vi "CRYAPI WSYSTEM MAIN.vi"(8 "sData":string, 9 "pVIF":refnum<vi>, 10 "sOption":string, 11 "sAction":string) -> (0 "bResult":bool=TRUE, 1 "pVIF_Out":refnum<vi>, 2 "sData_Out":string, 3 "tFrame_Out":T2)   [LabVIEW 2013]
uses:
  <vilib>/Utility/miscctls.llb/LVRectTypeDef.ctl
  CRYMain Sub Window Global.vi
  DataView/VIEW/CRYView Global.vi
  CRYProject/CRYProject Editor Global.vi
  DataView/VIEW/CRYNew View Global.vi
  CRYCurveLibrary/Global/CRYCurve Library Global.vi
  CRYStepSetup/CRYStepSetup Global.vi
  user32.dll
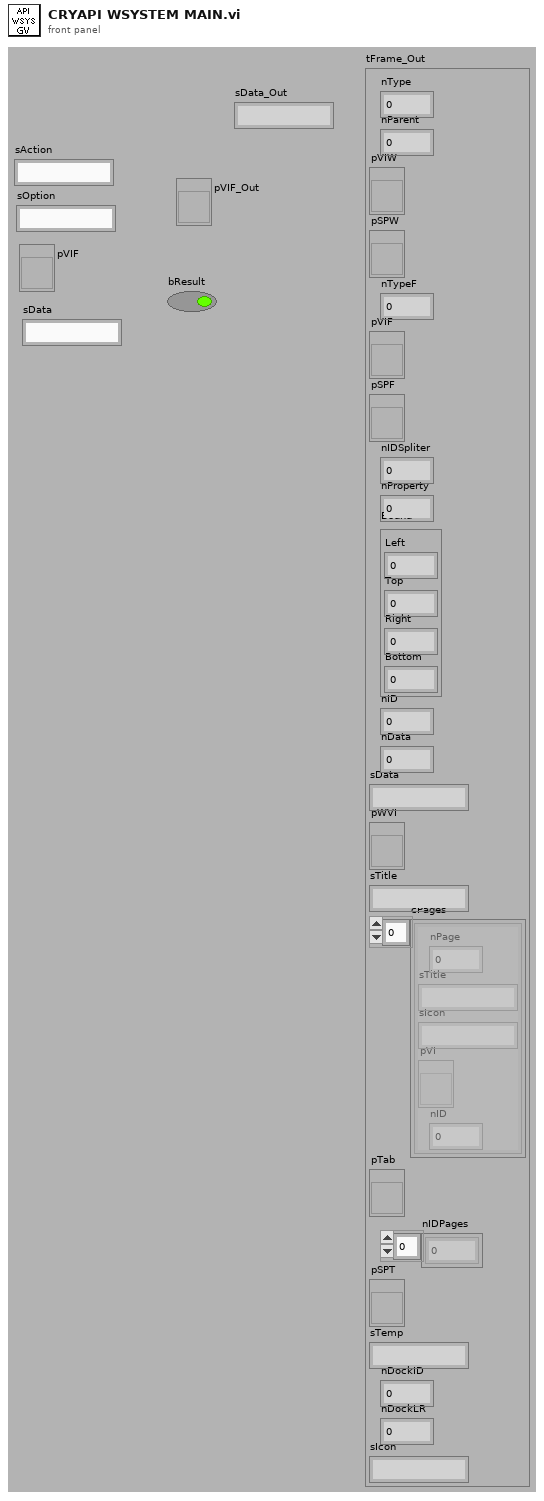
[diagram p1: front panel]
types:
  T1 = typedef "LVRectTypeDef.ctl" = cluster{"Left":i16, "Top":i16, "Right":i16, "Bottom":i16}
  T2 = cluster{"nType":i32, "nParent":i32, "pVIW":refnum<vi>, "pSPW":refnum<vi>, "nTypeF":i32, "pVIF":refnum<vi>, "pSPF":refnum<vi>, "nIDSpliter":i32, "nProperty":i32, "Bound":T1, "nID":i32, "nData":i32, "sData":string, "pWVI":refnum<vi>, "sTitle":string, "cPages":cluster{"nPage":i32, "sTitle":string, "sIcon":string, "pVI":refnum<vi>, "nID":i32}[], "pTab":refnum<vi>, "nIDPages":i32[], "pSPT":refnum<vi>, "sTemp":string, "nDockID":i32, "nDockLR":i32, "sIcon":string}
  T3 = enum32{"Invalid", "Standard", "Closed", "Hidden", "Minimized", "Maximized"}
  T4 = cluster{"nID":i32[], "Frame":cluster{"nType":i32, "nParent":i32, "pVIW":refnum<vi>, "pSPW":refnum<vi>, "nTypeF":i32, "pVIF":refnum<vi>, "pSPF":refnum<vi>, "nIDSpliter":i32, "nProperty":i32, "Bound":T1, "nID":i32, "nData":i32, "sData":string, "pWVI":refnum<vi>, "sTitle":string, "cPages":cluster{"nPage":i32, "sTitle":string, "sIcon":string, "pVI":refnum<vi>, "nID":i32}[], "pTab":refnum<vi>, "nIDPages":i32[], "pSPT":refnum<vi>, "sTemp":string, "nDockID":i32, "nDockLR":i32, "sIcon":string}[]}
  T5 = cluster{"nType":i32, "nParent":i32, "pVIW":refnum<vi>, "pSPW":refnum<vi>, "nTypeF":i32, "pVIF":refnum<vi>, "pSPF":refnum<vi>, "nIDSpliter":i32, "nProperty":i32, "Bound":T1, "nID":i32, "nData":i32, "sData":string, "pWVI":refnum<vi>, "sTitle":string, "cPages":cluster{"nPage":i32, "sTitle":string, "sIcon":string, "pVI":refnum<vi>, "nID":i32}[], "pTab":refnum<vi>, "nIDPages":i32[], "pSPT":refnum<vi>, "sTemp":string, "nDockID":i32, "nDockLR":i32, "sIcon":string}[]
  T6 = cluster{"Type Name":string, "Data Name":string, "Probe VIRef Number":i32, "Probe VIRef":refnum<vi>}[]
  T7 = cluster{"CLOSE_HIDE":i32, "CLOSE_CLOSE":i32, "DOCK_ENABLE":i32, "DOCK_DISABLE":i32, "FOCUS_SHOW":i32, "FOCUS_HIDE":i32}
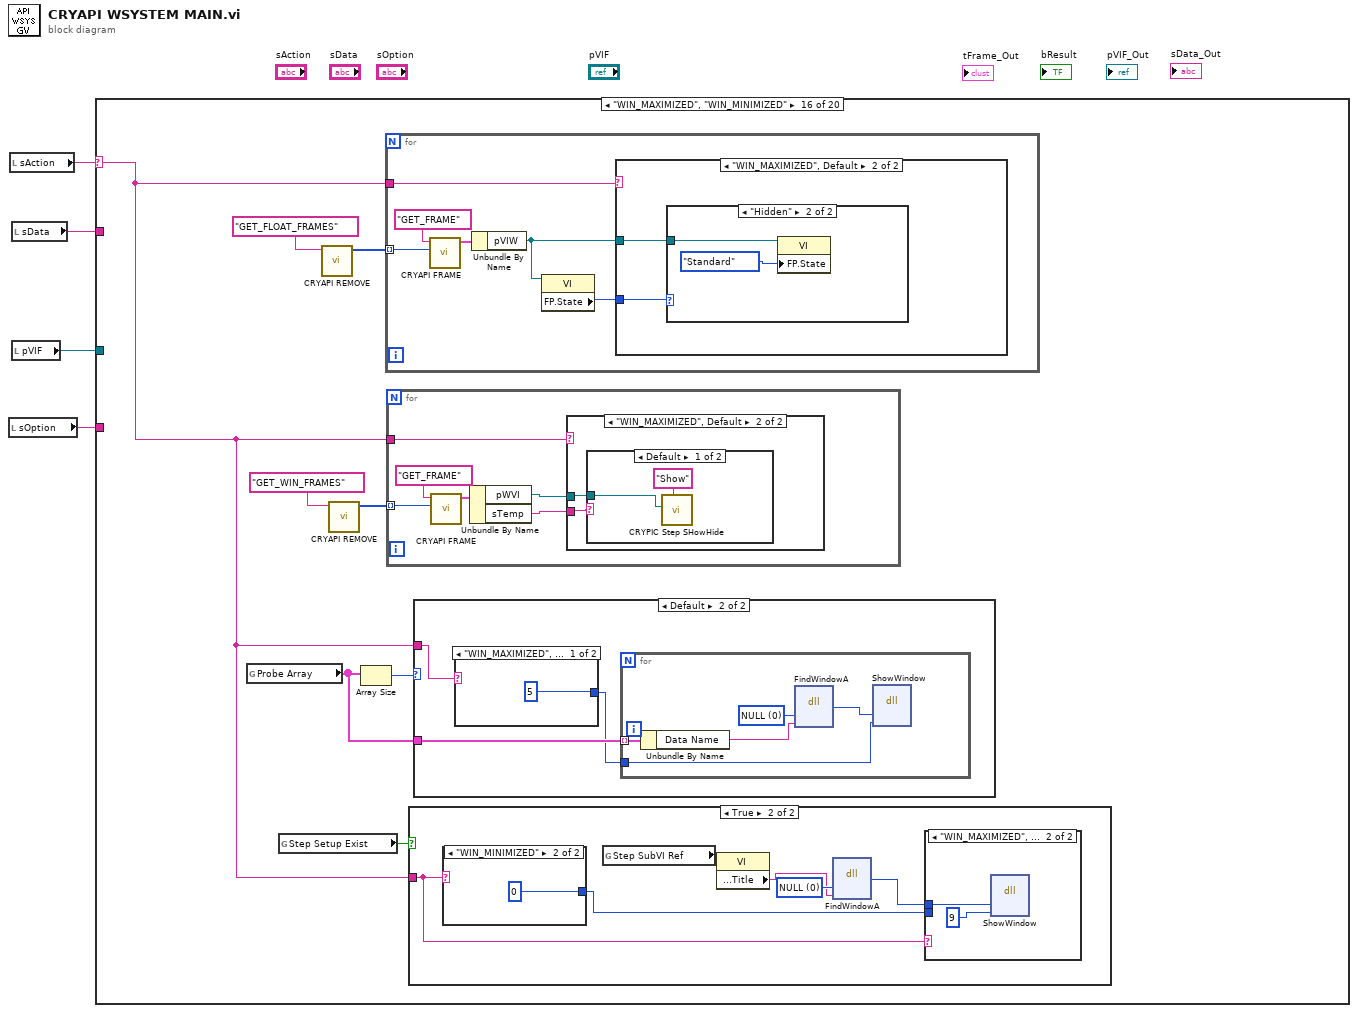
[diagram p0: block diagram]
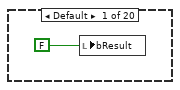
[diagram p2: hidden frame]
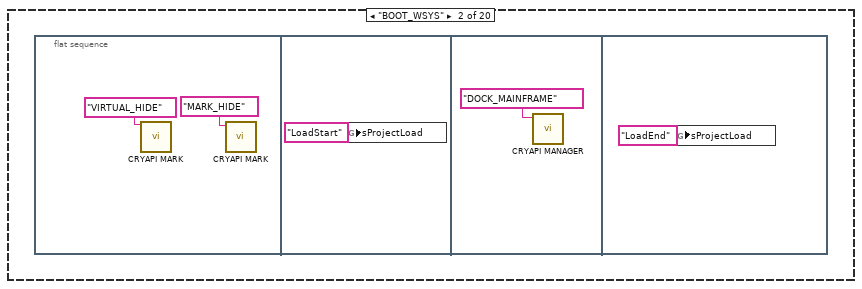
[diagram p3: hidden frame]
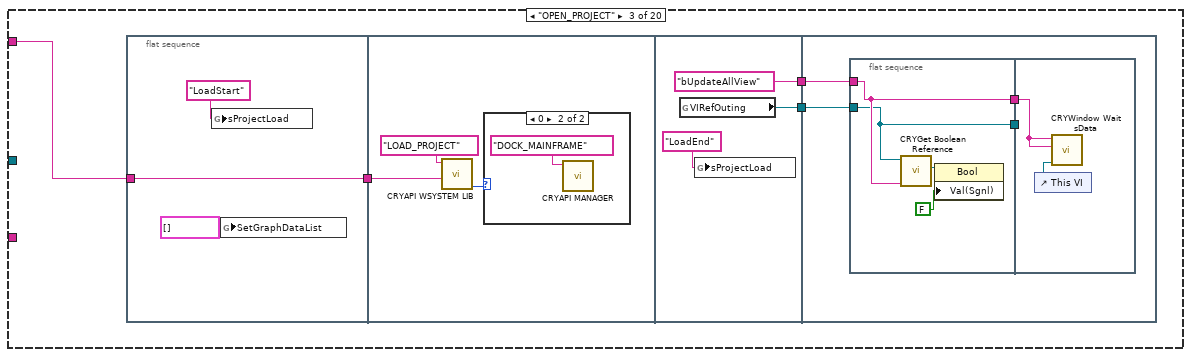
[diagram p4: hidden frame]
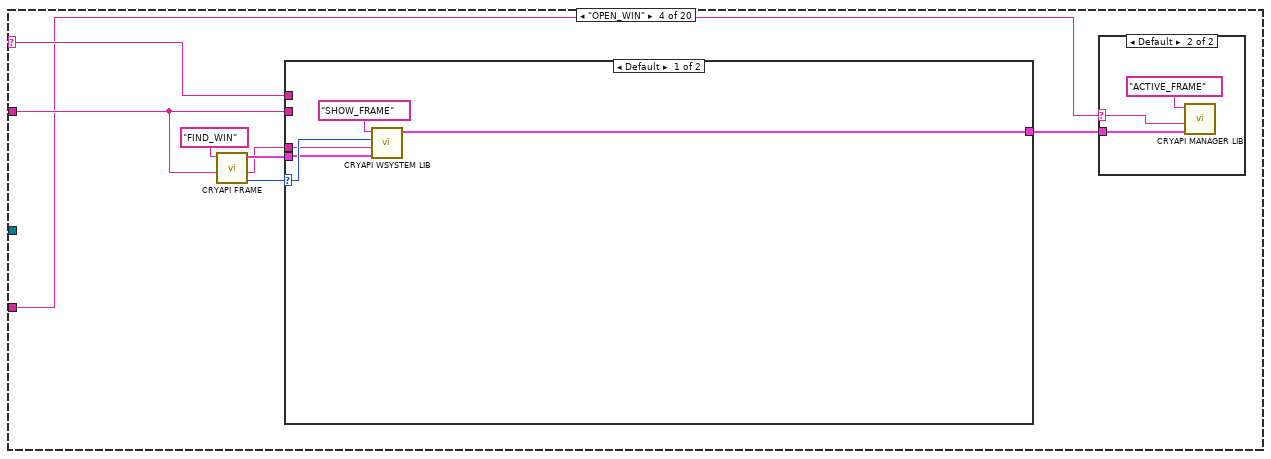
[diagram p6: hidden frame]
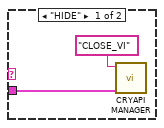
[diagram p7: hidden frame]
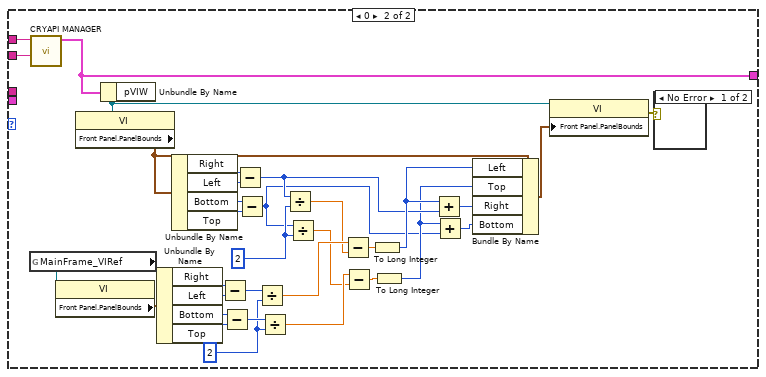
[diagram p8: hidden frame]
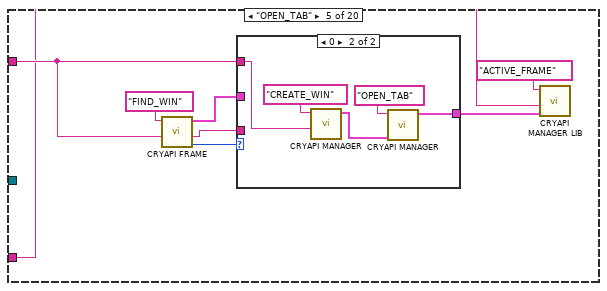
[diagram p10: hidden frame]
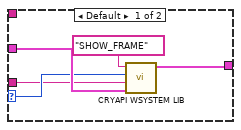
[diagram p11: hidden frame]
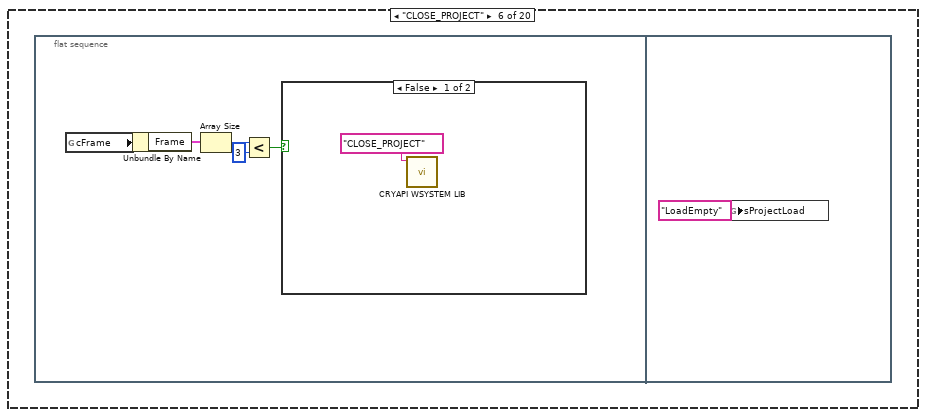
[diagram p12: hidden frame]
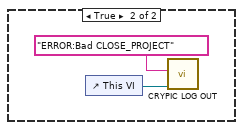
[diagram p13: hidden frame]
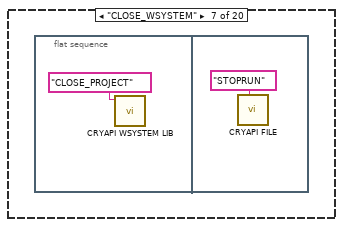
[diagram p14: hidden frame]
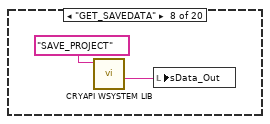
[diagram p15: hidden frame]
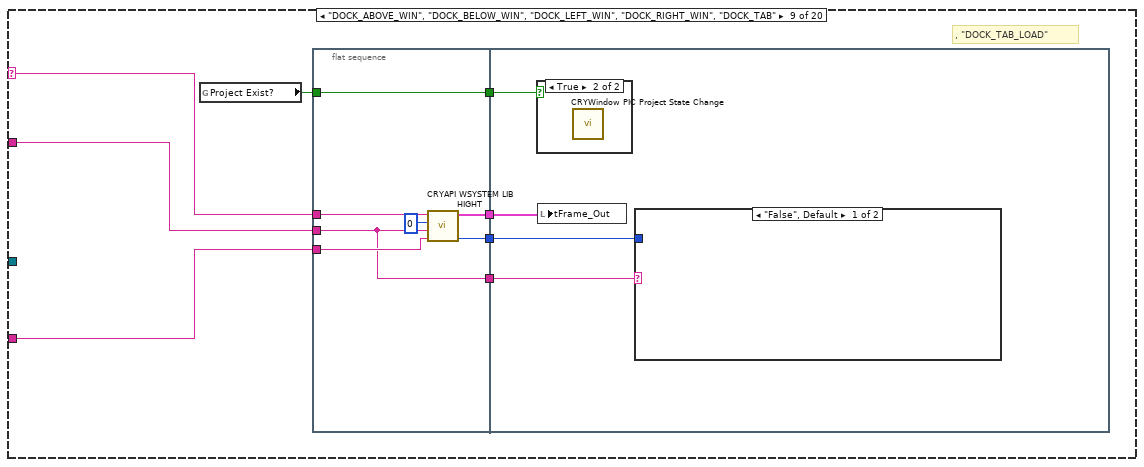
[diagram p16: hidden frame]
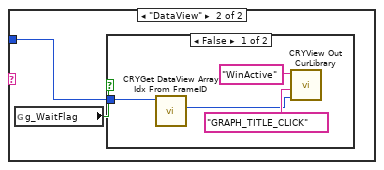
[diagram p17: hidden frame]
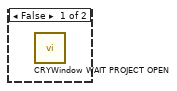
[diagram p19: hidden frame]
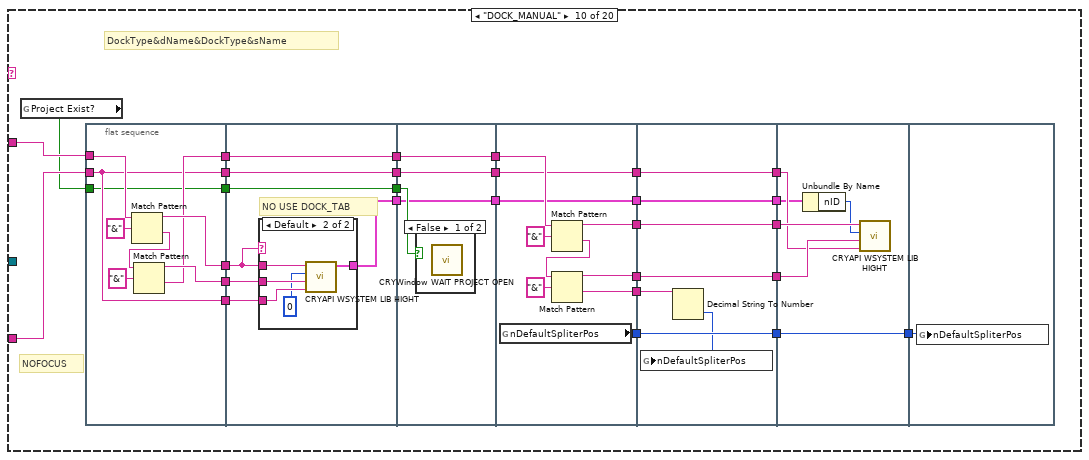
[diagram p20: hidden frame]
diagram:
  n1 = local read "sOption"() -> (w1:string)
  n2 = local read "sAction"() -> (w4:string)
  n3 = local read "sData"() -> (w3:string)
  n4 = local read "pVIF"() -> (w2:refnum<vi>)
  n5 = case shown="\"WIN_MAXIMIZED\", \"WIN_MINIMIZED\"" w4 {
    selector: w4 -> [_ _ _ w42 _ _ _ _ w122 _ _ w234 _ _ w292 w310 _ _ _ w422]
    tunnel: w3 -> [_ _ w14 w40 w90 _ _ _ w124 w165 _ w232 w275 w286 _ _ w375 w401 w420 _]
    tunnel: w2 -> [_ _ _ _ _ _ _ _ _ _ _ w241 _ _ _ _ _ _ _ _]
    tunnel: w1 -> [_ _ _ w35 w86 _ _ _ w123 w164 _ w230 w274 _ _ _ _ _ _ _]
    frame Default {
      n6 = local write "bResult"(FALSE) -> ()
    }
    frame "BOOT_WSYS" {
      n7 = flat-sequence {
        frame #0 {
          n8 = call "CRYAPI MARK.vi"("sAction"="VIRTUAL_HIDE") -> ()  [unwired: 3 in, 7 out]
          n9 = call "CRYAPI MARK.vi"("sAction"="MARK_HIDE") -> ()  [unwired: 3 in, 7 out]
        }
        frame #1 {
          n10 = global write "CRYMain Sub Window Global.vi" "sProjectLoad"("LoadStart" ("sProjectLoad")) -> ()
        }
        frame #2 {
          n11 = call "CRYAPI MANAGER.vi"("sAction"="DOCK_MAINFRAME") -> ()  [unwired: 4 in, 7 out]
        }
        frame #3 {
          n12 = global write "CRYMain Sub Window Global.vi" "sProjectLoad"("LoadEnd" ("sProjectLoad")) -> ()
        }
      }
    }
    frame "OPEN_PROJECT" {
      n13 = flat-sequence {
        tunnel: w14 -> [w17]
        tunnel: [w17] -> w13
        tunnel: w13 -> [w20]
        tunnel: ["bUpdateAllView" ("Label Name")] -> w12
        tunnel: [w22] -> w11
        tunnel: w12 -> [w26]
        tunnel: w11 -> [w25]
        frame #0 {
          n14 = global write "CRYMain Sub Window Global.vi" "sProjectLoad"("LoadStart" ("sProjectLoad")) -> ()
          n15 = global write "CRYView Global.vi" "SetGraphDataList"(cluster{"sAction":string, "sData":string}[] [] ("SetGraphDataList")) -> ()
        }
        frame #1 {
          n16 = call "CRYAPI WSYSTEM LIB.vi"("sData"=w20, "sAction"="LOAD_PROJECT") -> ("nData_Out"=w19:i32)  [unwired: 2 in, 7 out]
          n17 = case shown="0" w19 {
            frame Default {
            }
            frame 0 {
              n18 = call "CRYAPI MANAGER.vi"("sAction"="DOCK_MAINFRAME") -> ()  [unwired: 4 in, 7 out]
            }
          }
        }
        frame #2 {
          n19 = global read "CRYView Global.vi" "VIRefOuting"() -> (w22:refnum<vi>)
          n20 = global write "CRYMain Sub Window Global.vi" "sProjectLoad"("LoadEnd" ("sProjectLoad")) -> ()
        }
        frame #3 {
          n21 = flat-sequence {
            tunnel: [w29] -> w28
            tunnel: [w30] -> w27
            tunnel: w26 -> [w30]
            tunnel: w25 -> [w29]
            tunnel: w28 -> [_]
            tunnel: w27 -> [w33]
            frame #0 {
              n22 = call "CRYGet Boolean Reference.vi"("Label Name"=w30, "VI Refnum"=w29) -> ("Boolean Ref"=w32:refnum<vi>)  [unwired: 7 in, 2 out]
              n23 = property class="Bool"(reference=w32, "Val(Sgnl)"=FALSE) -> ()  [unwired: 1 in, 2 out]
            }
            frame #1 {
              n24 = control-ref of="This VI"() -> (w34:refnum<vi>)
              n25 = call "CRYWindow Wait sData.vi"("pVIRef"=w34, "sData"=w33, "sAction"=w33) -> ()  [unwired: 8 in, 1 out]
            }
          }
        }
      }
    }
    frame "OPEN_WIN" {
      n26 = call "CRYAPI FRAME.vi"("sData"=w40, "sAction"="FIND_WIN") -> ("nData_Out"=w39:i32, "sData_Out"=w36:string, "tFrame_Out"=w38:T2)  [unwired: 4 in, 3 out]
      n27 = case shown="Default" w39 {
        selector: w39 -> [w51 _]
        tunnel: w40 -> [_ w85]
        tunnel: w42 -> [_ w84]
        tunnel: w38 -> [w50 _]
        tunnel: [w49 w83] -> w37
        tunnel: w36 -> [w48 _]
        frame Default {
          n28 = call "CRYAPI WSYSTEM LIB.vi"("tFrame"=w50, "sData"=w48, "nData"=w51, "sAction"="SHOW_FRAME") -> ("tFrame_Out"=w49:T2)  [unwired: 7 out]
        }
        frame 0 {
          w69 = 2
          w70 = 2
          n29 = global read "CRYMain Sub Window Global.vi" "MainFrame_VIRef"() -> (w73:refnum<vi>)
          n30 = call "CRYAPI MANAGER.vi"("sData"=w85, "sAction"=w84) -> ("tFrame_Out"=w83:T2)  [unwired: 3 in, 6 out]
          n31 = property class="VI"(reference=w73) -> ("Front Panel.PanelBounds"=w74:T1)  [unwired: 1 in, 2 out]
          n32 = Unbundle By Name(w83) -> ("pVIW"=w62:refnum<vi>)
          n33 = property class="VI"(reference=w62) -> ("Front Panel.PanelBounds"=w61:T1)  [unwired: 1 in, 2 out]
          n34 = Unbundle By Name(w74) -> ("Right"=w76:i16, "Left"=w75:i16, "Bottom"=w77:i16, "Top"=w78:i16)
          n35 = Unbundle By Name(w61) -> ("Right"=w81:i16, "Left"=w82:i16, "Bottom"=w80:i16, "Top"=w79:i16)
          n36 = Subtract(x=w76, y=w75) -> (x-y=w72:i16)
          n37 = Subtract(x=w77, y=w78) -> (x-y=w71:i16)
          n38 = Subtract(x=w81, y=w82) -> (x-y=w58:i16)
          n39 = Subtract(x=w80, y=w79) -> (x-y=w55:i16)
          n40 = Divide(x=w72, y=w70) -> (x/y=w68:dbl)
          n41 = Divide(x=w71, y=w70) -> (x/y=w66:dbl)
          n42 = Divide(x=w58, y=w69) -> (x/y=w67:dbl)
          n43 = Divide(x=w55, y=w69) -> (x/y=w65:dbl)
          n44 = Subtract(x=w68, y=w67) -> (x-y=w64:dbl)
          n45 = Subtract(x=w66, y=w65) -> (x-y=w63:dbl)
          n46 = To Long Integer(number=w64) -> (32bit integer=w59:i32)
          n47 = To Long Integer(number=w63) -> (32bit integer=w56:i32)
          n48 = Add(x=w59, y=w58) -> (x+y=w60:i32)
          n49 = Add(x=w56, y=w55) -> (x+y=w57:i32)
          n50 = Bundle By Name(cluster=w61, "Left"=w59, "Top"=w56, "Right"=w60, "Bottom"=w57) -> (w54:T1)
          n51 = property class="VI"(reference=w62, "Front Panel.PanelBounds"=w54) -> (error out=w53:errorcluster)  [unwired: 1 in, 1 out]
          n52 = case shown="No Error" w53 {
            frame No Error {
            }
            frame Error {
            }
          }
        }
      }
      n53 = case shown="Default" w35 {
        selector: w35 -> [_ w45]
        tunnel: w37 -> [w43 w47]
        frame "HIDE" {
          n54 = call "CRYAPI MANAGER.vi"("tFrame"=w43, "sAction"="CLOSE_VI") -> ()  [unwired: 3 in, 7 out]
        }
        frame Default {
          n55 = call "CRYAPI MANAGER LIB.vi"("tFrame"=w47, "sData"=w45, "sAction"="ACTIVE_FRAME") -> ()  [unwired: 6 in, 3 out]
        }
      }
    }
    frame "OPEN_TAB" {
      n56 = call "CRYAPI FRAME.vi"("sData"=w90, "sAction"="FIND_WIN") -> ("nData_Out"=w92:i32, "sData_Out"=w87:string, "tFrame_Out"=w91:T2)  [unwired: 4 in, 3 out]
      n57 = case shown="0" w92 {
        selector: w92 -> [w96 _]
        tunnel: w91 -> [w97 _]
        tunnel: w90 -> [_ w100]
        tunnel: [w95 w99] -> w88
        tunnel: w87 -> [w94 _]
        frame Default {
          n58 = call "CRYAPI WSYSTEM LIB.vi"("tFrame"=w97, "sData"=w94, "nData"=w96, "sAction"="SHOW_FRAME") -> ("tFrame_Out"=w95:T2)  [unwired: 7 out]
        }
        frame 0 {
          n59 = call "CRYAPI MANAGER.vi"("sData"=w100, "sAction"="CREATE_WIN") -> ("tFrame_Out"=w101:T2)  [unwired: 3 in, 6 out]
          n60 = call "CRYAPI MANAGER.vi"("tFrame"=w101, "sAction"="OPEN_TAB") -> ("tFrame_Out"=w99:T2)  [unwired: 3 in, 6 out]
        }
      }
      n61 = call "CRYAPI MANAGER LIB.vi"("tFrame"=w88, "sData"=w86, "sAction"="ACTIVE_FRAME") -> ()  [unwired: 6 in, 3 out]
    }
    frame "CLOSE_PROJECT" {
      n62 = flat-sequence {
        frame #0 {
          n63 = global read "CRYMain Sub Window Global.vi" "cFrame"() -> (w108:T4)
          n64 = Unbundle By Name(w108) -> ("Frame"=w107:T5)
          n65 = Array Size(array=w107) -> (size(s)=w106:i32)
          n66 = Less?(x=w106, y=3) -> (x < y?=w104:bool)
          n67 = case shown="False" w104 {
            frame False {
              n68 = call "CRYAPI WSYSTEM LIB.vi"("sAction"="CLOSE_PROJECT") -> ()  [unwired: 3 in, 8 out]
            }
            frame True {
              n69 = control-ref of="This VI"() -> (w110:refnum<vi>)
              n70 = call "CRYPIC LOG OUT.vi"("pVIRef"=w110, "sData"="ERROR:Bad CLOSE_PROJECT") -> ()  [unwired: 10 in]
            }
          }
        }
        frame #1 {
          n71 = global write "CRYMain Sub Window Global.vi" "sProjectLoad"("LoadEmpty" ("sProjectLoad")) -> ()
        }
      }
    }
    frame "CLOSE_WSYSTEM" {
      n72 = flat-sequence {
        frame #0 {
          n73 = call "CRYAPI WSYSTEM LIB.vi"("sAction"="CLOSE_PROJECT") -> ()  [unwired: 3 in, 8 out]
        }
        frame #1 {
          n74 = call "CRYAPI FILE.vi"("sAction"="STOPRUN") -> ()  [unwired: 3 in, 8 out]
        }
      }
    }
    frame "GET_SAVEDATA" {
      n75 = call "CRYAPI WSYSTEM LIB.vi"("sAction"="SAVE_PROJECT") -> ("sData_Out"=w115:string)  [unwired: 3 in, 7 out]
      n76 = local write "sData_Out"(w115) -> ()
    }
    frame "DOCK_ABOVE_WIN", "DOCK_BELOW_WIN", "DOCK_LEFT_WIN", "DOCK_RIGHT_WIN", "DOCK_TAB" {
      # ", \"DOCK_TAB_LOAD\""
      n77 = global read "CRYProject Editor Global.vi" "Project Exist?"() -> (w119:bool)
      n78 = flat-sequence {
        tunnel: [w127] -> w121
        tunnel: [w128] -> w120
        tunnel: w124 -> [w126]
        tunnel: w123 -> [w131]
        tunnel: w122 -> [w130]
        tunnel: w119 -> [w127]
        tunnel: [w126] -> w118
        tunnel: [w125] -> w117
        tunnel: w121 -> [w135]
        tunnel: w120 -> [w134]
        tunnel: w118 -> [w133]
        tunnel: w117 -> [w132]
        frame #0 {
          n79 = call "CRYAPI WSYSTEM LIB HIGHT.vi"("sOption"=w131, "sData"=w126, "nData"=0, "sAction"=w130) -> ("nData_Out"=w125:i32, "tFrame_Out"=w128:T2)  [unwired: 6 out]
        }
        frame #1 {
          n80 = case shown="True" w135 {
            frame False {
              n81 = call "CRYWindow WAIT PROJECT OPEN.vi"() -> ()  [unwired: 12 in]
            }
            frame True {
              n82 = call "CRYWindow PIC Project State Change.vi"() -> ()  [unwired: 12 in]
            }
          }
          n83 = local write "tFrame_Out"(w134) -> ()
          n84 = case shown="\"False\", Default" w133 {
            tunnel: w132 -> [_ w137]
            frame "False", Default {
            }
            frame "DataView" {
              n85 = global read "CRYNew View Global.vi" "g_WaitFlag"() -> (w136:bool)
              n86 = case shown="False" w136 {
                tunnel: w137 -> [w138 _]
                frame False {
                  n87 = call "CRYGet DataView Array Idx From FrameID.vi"("Frame nID"=w138) -> ("DataView idx"=w139:i32)  [unwired: 9 in, 1 out]
                  n88 = call "CRYView Out CurLibrary.vi"("DataView Idx"=w139, "sData"="GRAPH_TITLE_CLICK", "sAction"="WinActive") -> ()  [unwired: 7 in, 2 out]
                }
                frame True {
                }
              }
            }
          }
        }
      }
    }
    frame "DOCK_MANUAL" {
      # "NOFOCUS"
      # "DockType&dName&DockType&sName"
      n89 = global read "CRYProject Editor Global.vi" "Project Exist?"() -> (w163:bool)
      n90 = flat-sequence {
        tunnel: [w174] -> w169
        tunnel: [w175] -> w168
        tunnel: [w173] -> w166
        tunnel: w165 -> [w172]
        tunnel: w164 -> [w171]
        tunnel: w163 -> [w170]
        tunnel: [w171] -> w162
        tunnel: [w171] -> w161
        tunnel: [w170] -> w160
        tunnel: w169 -> [w185]
        tunnel: w168 -> [w184]
        tunnel: [w183] -> w167
        tunnel: w166 -> [w183]
        tunnel: w162 -> [w179]
        tunnel: w161 -> [w182]
        tunnel: w160 -> [w181]
        tunnel: [w181] -> w159
        tunnel: [w180] -> w156
        tunnel: [w179] -> w154
        tunnel: w167 -> [w198]
        tunnel: w159 -> [w197]
        tunnel: [w198] -> w158
        tunnel: [w196] -> w157
        tunnel: w156 -> [w196]
        tunnel: [w195] -> w155
        tunnel: w154 -> [w195]
        tunnel: w158 -> [w207]
        tunnel: w157 -> [w205]
        tunnel: [w206] -> w153
        tunnel: [w201] -> w151
        tunnel: [w205] -> w149
        tunnel: w155 -> [w204]
        tunnel: [w204] -> w147
        tunnel: [w200] -> w145
        tunnel: [w199] -> w144
        tunnel: w153 -> [w215]
        tunnel: [w215] -> w152
        tunnel: w151 -> [w214]
        tunnel: [w214] -> w150
        tunnel: w149 -> [w213]
        tunnel: [w213] -> w148
        tunnel: w147 -> [w212]
        tunnel: [w212] -> w146
        tunnel: w145 -> [w210]
        tunnel: w144 -> [w211]
        tunnel: [w211] -> w142
        tunnel: w152 -> [w221]
        tunnel: w150 -> [w220]
        tunnel: w148 -> [w216]
        tunnel: w146 -> [w219]
        tunnel: [w217] -> w143
        tunnel: w142 -> [w217]
        tunnel: w143 -> [w222]
        frame #0 {
          n91 = Match Pattern(string=w172, regular expression="&") -> (before substring=w175:string, after substring=w177:string)  [unwired: 1 in, 2 out]
          n92 = Match Pattern(string=w177, regular expression="&") -> (before substring=w174:string, after substring=w173:string)  [unwired: 1 in, 2 out]
        }
        frame #1 {
          # "NO USE DOCK_TAB"
          n93 = case shown="Default" w184 {
            tunnel: w184 -> [w188 w194]
            tunnel: w185 -> [w187 w193]
            tunnel: w182 -> [_ w192]
            tunnel: [w186 w191] -> w180
            frame "DOCK_TAB" {
              n94 = call "CRYAPI WSYSTEM LIB HIGHT.vi"("sData"=w187, "nData"=0, "sAction"=w188) -> ("tFrame_Out"=w186:T2)  [unwired: 1 in, 7 out]
            }
            frame Default {
              n95 = call "CRYAPI WSYSTEM LIB HIGHT.vi"("sOption"=w192, "sData"=w193, "nData"=0, "sAction"=w194) -> ("tFrame_Out"=w191:T2)  [unwired: 7 out]
            }
          }
        }
        frame #2 {
          n96 = case shown="False" w197 {
            frame False {
              n97 = call "CRYWindow WAIT PROJECT OPEN.vi"() -> ()  [unwired: 12 in]
            }
            frame True {
              n98 = call "CRYWindow PIC Project State Change.vi"() -> ()  [unwired: 12 in]
            }
          }
        }
        frame #3 {
          n99 = global read "CRYMain Sub Window Global.vi" "nDefaultSpliterPos"() -> (w199:i32)
          n100 = Match Pattern(string=w207, regular expression="&") -> (before substring=w206:string, after substring=w202:string)  [unwired: 1 in, 2 out]
          n101 = Match Pattern(string=w202, regular expression="&") -> (before substring=w201:string, after substring=w200:string)  [unwired: 1 in, 2 out]
        }
        frame #4 {
          n102 = Decimal String To Number(string=w210) -> (number=w209:i32)  [unwired: 2 in, 1 out]
          n103 = global write "CRYMain Sub Window Global.vi" "nDefaultSpliterPos"(w209) -> ()
        }
        frame #5 {
          n104 = Unbundle By Name(w216) -> ("nID"=w218:i32)
          n105 = call "CRYAPI WSYSTEM LIB HIGHT.vi"("sOption"=w219, "sData"=w220, "nData"=w218, "sAction"=w221) -> ()  [unwired: 8 out]
        }
        frame #6 {
          n106 = global write "CRYMain Sub Window Global.vi" "nDefaultSpliterPos"(w222) -> ()
        }
      }
    }
    frame "LOAD_MARK" {
      n107 = call "CRYAPI LOAD.vi"("sAction"="LOAD_MARK") -> ()  [unwired: 5 in, 6 out]
    }
    frame "GET_SUBREF", "SET_SUBREF-----", "SET_SUBREF_ORG----", "SET_SUBREF_TEST" {
      n108 = call "CRYAPI FRAME.vi"("sData"=w232, "sAction"="FIND_WIN") -> ("nData_Out"=w237:i32, "sData_Out"=w239:string, "tFrame_Out"=w238:T2)  [unwired: 4 in, 3 out]
      n109 = case shown="Default" w237 {
        selector: w237 -> [w258 _]
        tunnel: w232 -> [w254 w272]
        tunnel: w234 -> [w253 w270]
        tunnel: w238 -> [w257 _]
        tunnel: [w256 w273] -> w231
        tunnel: w239 -> [w255 _]
        tunnel: [w254 w272] -> w235
        tunnel: [w252 w270] -> w225
        tunnel: w230 -> [w251 w269]
        tunnel: [w250 w269] -> w229
        frame Default {
          n110 = case shown="Default" w253 {
            selector: w253 -> [w259 w263]
            tunnel: w258 -> [_ w267]
            tunnel: w257 -> [w261 w266]
            tunnel: [w261 w265] -> w256
            tunnel: w255 -> [_ w264]
            tunnel: [w259 w263] -> w252
            tunnel: w251 -> [w260 w262]
            tunnel: [w260 w262] -> w250
            frame "SET_SUBREF_ORG" {
            }
            frame Default {
              n111 = call "CRYAPI WSYSTEM LIB.vi"("tFrame"=w266, "sData"=w264, "nData"=w267, "sAction"="SHOW_FRAME") -> ("tFrame_Out"=w265:T2)  [unwired: 7 out]
            }
          }
        }
        frame 0 {
          n112 = call "CRYAPI MANAGER.vi"("sData"=w272, "sAction"="OPEN_WIN") -> ("tFrame_Out"=w273:T2)  [unwired: 3 in, 6 out]
        }
      }
      n113 = Bundle By Name(cluster=w231, "pWVI"=w241) -> (w240:T2)
      n114 = case shown="\"SET_SUBREF\"" w225 {
        selector: w225 -> [w243 w245 _]
        tunnel: w231 -> [_ w248 _]
        tunnel: [_ w247 _] -> w233
        tunnel: w229 -> [_ w246 _]
        tunnel: [w243 w245 "SET_SUBREF"] -> w228
        frame "False", Default {
        }
        frame "SET_SUBREF" {
          n115 = call "CRYAPI MANAGER LIB.vi"("tFrame"=w248, "sData"=w246, "sAction"="ACTIVE_FRAME") -> ("nData_Out"=w247:i32)  [unwired: 6 in, 2 out]
        }
        frame "SET_SUBREF_ORG" {
        }
      }
      n116 = call "CRYAPI WSYSTEM LIB.vi"("tFrame"=w240, "sData"=w235, "nData"=w233, "sAction"=w228) -> ("tFrame_Out"=w224:T2)  [unwired: 7 out]
      n117 = Unbundle By Name(w224) -> ("nData"=w226:i32)
      n118 = Unbundle By Name(w224) -> ("pWVI"=w242:refnum<vi>)
      n119 = Greater Than 0?(x=w226) -> (x > 0?=w227:bool)
      n120 = local write "pVIF_Out"(w242) -> ()
      n121 = local write "bResult"(w227) -> ()
    }
    frame "LOAD_DOC" {
      n122 = Empty String/Path?(string/path=w275) -> (empty?=w276:bool)
      n123 = case shown="False" w276 {
        tunnel: w275 -> [w279 _]
        tunnel: w274 -> [w278 _]
        frame False {
          n124 = call "CRYAPI MANAGER LIB.vi"("sOption"=w278, "sData"=w279, "sAction"="LOAD_DOC") -> ("nData_Out"=w277:i32)  [unwired: 2 in, 6 out]
          n125 = case shown="1" w277 {
            selector: w277 -> [_ w281]
            frame 0, Default {
            }
            frame 1 {
              n126 = call "CRYAPI WSYSTEM LIB HIGHT.vi"("sData"="Project Document" ("sAction"), "nData"=w281, "sAction"="DOCK_TAB") -> ()  [unwired: 1 in, 8 out]
            }
          }
        }
        frame True {
        }
      }
    }
    frame "SAVE_DOC" {
      n127 = call "CRYAPI MANAGER LIB.vi"("sData"=w286, "sAction"="SAVE_DOC") -> ("sData_Out"=w284:string)  [unwired: 3 in, 6 out]
      n128 = local write "sData_Out"(w284) -> ()
    }
    frame "ISDOCUMENT", "PAGESETUP", "PRINT" {
      n129 = call "CRYAPI FRAME.vi"("sData"="Document" ("sAction"), "sAction"="FIND_WIN") -> ("nData_Out"=w289:i32, "sData_Out"=w288:string, "tFrame_Out"=w287:T2)  [unwired: 4 in, 3 out]
      n130 = case shown="\"PAGESETUP\", \"PRINT\", Default" w292 {
        selector: w292 -> [w301 _]
        tunnel: w289 -> [_ _]
        tunnel: w288 -> [_ w307]
        tunnel: w287 -> [_ _]
        frame "PAGESETUP", "PRINT", Default {
          n131 = call "CRYAPI WSYSTEM LIB HIGHT.vi"("sData"="Document" ("Window Type"), "nData"=0, "sAction"="DOCK_TAB") -> ("tFrame_Out"=w296:T2)  [unwired: 1 in, 7 out]
          n132 = case shown="\"PAGESETUP\"" w301 {
            tunnel: ["" ("Label Name") "BtnPage" ("Label Name") "BtnPrint" ("Label Name")] -> w299
            frame Default {
            }
            frame "PAGESETUP" {
            }
            frame "PRINT" {
            }
          }
          n133 = Unbundle By Name(w296) -> ("pWVI"=w300:refnum<vi>)
          n134 = call "CRYGet Boolean Reference.vi"("Label Name"=w299, "VI Refnum"=w300) -> ("Exist?"=w298:bool, "Boolean Ref"=w297:refnum<vi>)  [unwired: 8 out]
          n135 = case shown="True" w298 {
            tunnel: w297 -> [_ w303]
            frame False {
            }
            frame True {
              n136 = property class="Bool"(reference=w303, "Val(Sgnl)"=TRUE) -> ()  [unwired: 1 in, 2 out]
            }
          }
        }
        frame "ISDOCUMENT" {
          n137 = case shown="\"OPEN\"" w307 {
            frame Default {
              n138 = local write "bResult"(FALSE ("bResult")) -> ()
            }
            frame "OPEN" {
              n139 = local write "bResult"(TRUE ("bResult")) -> ()
            }
          }
        }
      }
    }
    frame "WIN_MAXIMIZED", "WIN_MINIMIZED" {
      n140 = global read "CRYCurve Library Global.vi" "Probe Array"() -> (w312:T6)
      n141 = global read "CRYStepSetup Global.vi" "Step Setup Exist"() -> (w311:bool)
      n142 = call "CRYAPI REMOVE.vi"("sAction"="GET_FLOAT_FRAMES") -> ("List_ID_Out"=w317:i32[])  [unwired: 4 in, 6 out]
      n143 = call "CRYAPI REMOVE.vi"("sAction"="GET_WIN_FRAMES") -> ("List_ID_Out"=w314:i32[])  [unwired: 4 in, 6 out]
      n144 = Array Size(array=w312) -> (size(s)=w313:i32)
      n145 = for {
        tunnel: w317 -> [w359] mode=indexing
        tunnel: w310 -> [w357]
        n146 = call "CRYAPI FRAME.vi"("nData"=w359, "sAction"="GET_FRAME") -> ("tFrame_Out"=w354:T2)  [unwired: 4 in, 5 out]
        n147 = Unbundle By Name(w354) -> ("pVIW"=w355:refnum<vi>)
        n148 = property class="VI"(reference=w355) -> ("FP.State"=w356:T3)  [unwired: 1 in, 2 out]
        n149 = case shown="\"WIN_MAXIMIZED\", Default" w357 {
          tunnel: w356 -> [w361 w365]
          tunnel: w355 -> [w360 w364]
          frame "WIN_MINIMIZED" {
            n150 = case shown="\"Standard\"" w361 {
              tunnel: w360 -> [_ w363]
              frame "Invalid", Default {
              }
              frame "Standard" {
                n151 = property class="VI"(reference=w363, "FP.State"=T3."Hidden" ("Front Panel Window:State")) -> ()  [unwired: 1 in, 2 out]
              }
            }
          }
          frame "WIN_MAXIMIZED", Default {
            n152 = case shown="\"Hidden\"" w365 {
              tunnel: w364 -> [_ w367]
              frame "Invalid", Default {
              }
              frame "Hidden" {
                n153 = property class="VI"(reference=w367, "FP.State"=T3."Standard" ("Front Panel Window:State")) -> ()  [unwired: 1 in, 2 out]
              }
            }
          }
        }
      }
      n154 = for {
        tunnel: w314 -> [w345] mode=indexing
        tunnel: w310 -> [w343]
        n155 = call "CRYAPI FRAME.vi"("nData"=w345, "sAction"="GET_FRAME") -> ("tFrame_Out"=w341:T2)  [unwired: 4 in, 5 out]
        n156 = Unbundle By Name(w341) -> ("pWVI"=w342:refnum<vi>, "sTemp"=w340:string)
        n157 = case shown="\"WIN_MAXIMIZED\", Default" w343 {
          tunnel: w342 -> [w347 w351]
          tunnel: w340 -> [w346 w350]
          frame "WIN_MINIMIZED" {
            n158 = case shown="Default" w346 {
              tunnel: w347 -> [w348 _]
              frame Default {
                n159 = call "CRYPIC Step SHowHide.vi"("sAction"="Hide", "VIRef"=w348) -> ()  [unwired: 10 in]
              }
              frame "Step Setup" {
              }
            }
          }
          frame "WIN_MAXIMIZED", Default {
            n160 = case shown="Default" w350 {
              tunnel: w351 -> [w352 _]
              frame Default {
                n161 = call "CRYPIC Step SHowHide.vi"("sAction"="Show", "VIRef"=w352) -> ()  [unwired: 10 in]
              }
              frame "Step Setup" {
              }
            }
          }
        }
      }
      n162 = case shown="True" w311 {
        tunnel: w310 -> [_ w319]
        frame False {
        }
        frame True {
          w322 = 0 items=["NULL"]
          n163 = case shown="\"WIN_MINIMIZED\"" w319 {
            tunnel: [5 ("nCmdShow") 0 ("nCmdShow")] -> w318
            frame "WIN_MAXIMIZED", Default {
            }
            frame "WIN_MINIMIZED" {
            }
          }
          n164 = global read "CRYStepSetup Global.vi" "Step SubVI Ref"() -> (w323:refnum<vi>)
          n165 = property class="VI"(reference=w323) -> ("Front Panel.Title"=w321:string)  [unwired: 1 in, 2 out]
          n166 = dll-call lib="user32.dll" fn="FindWindowA" label="FindWindow"("lpszClassName"=w322, "lpszWindowName"=w321) -> ("hWnd"=w320:u32)  [unwired: 4 in, 3 out]
          n167 = case shown="\"WIN_MAXIMIZED\", Default" w319 {
            tunnel: w320 -> [w325 w327]
            tunnel: w318 -> [w324 _]
            frame "WIN_MINIMIZED" {
              n168 = dll-call lib="user32.dll" fn="ShowWindow"("Handle"=w325, "nCmdShow"=w324) -> ()  [unwired: 5 in, 3 out]
            }
            frame "WIN_MAXIMIZED", Default {
              n169 = dll-call lib="user32.dll" fn="ShowWindow"("Handle"=w327, "nCmdShow"=9) -> ()  [unwired: 5 in, 3 out]
            }
          }
        }
      }
      n170 = case shown="Default" w313 {
        tunnel: w310 -> [_ w332]
        tunnel: w312 -> [_ w331]
        frame 0 {
        }
        frame Default {
          n171 = case shown="\"WIN_MAXIMIZED\", Default" w332 {
            tunnel: [5 ("nCmdShow") 0 ("nCmdShow")] -> w330
            frame "WIN_MAXIMIZED", Default {
            }
            frame "WIN_MINIMIZED" {
            }
          }
          n172 = for {
            tunnel: w331 -> [w337] mode=indexing
            tunnel: w330 -> [w333]
            w335 = 0 items=["NULL"]
            n173 = Unbundle By Name(w337) -> ("Data Name"=w334:string)
            n174 = dll-call lib="user32.dll" fn="FindWindowA" label="FindWindow"("lpszClassName"=w335, "lpszWindowName"=w334) -> ("hWnd"=w336:u32)  [unwired: 4 in, 3 out]
            n175 = dll-call lib="user32.dll" fn="ShowWindow"("Handle"=w336, "nCmdShow"=w333) -> ()  [unwired: 5 in, 3 out]
          }
        }
      }
    }
    frame "CloseStepView" {
      n176 = Match Pattern(string=w375, regular expression="&T&") -> (before substring=w374:string, after substring=w369:string)  [unwired: 1 in, 2 out]
      n177 = call "CRYPIC PreGetVIName.vi"("sVIName"=w374) -> ("sVIName_Out"=w368:string)  [unwired: 9 in, 1 out]
      n178 = call "CRYAPI MANAGER LIB.vi"("sOption"=w374, "sData"=w368, "sAction"="FIND_WINDOW") -> ("nData_Out"=w371:i32, "tFrame_Out"=w373:T2)  [unwired: 6 in, 1 out]
      n179 = case shown="Default" w371 {
        selector: w371 -> [w379 _]
        tunnel: w373 -> [w378 _]
        tunnel: [w378 w380] -> w372
        tunnel: [w379 w381] -> w370
        tunnel: w369 -> [_ w384]
        frame Default {
        }
        frame 0 {
          n180 = call "CRYConvert ASCII to Unicode.vi"("ASCII"=w384) -> ("Unicode"=w383:string)  [unwired: 4 in]
          n181 = call "CRYAPI MANAGER LIB.vi"("sOption"="StepView", "sData"=w383, "sAction"="FIND_WINDOW") -> ("nData_Out"=w381:i32, "tFrame_Out"=w380:T2)  [unwired: 6 in, 1 out]
        }
      }
      n182 = case shown="Default" w370 {
        tunnel: w372 -> [w387 _]
        frame Default {
          n183 = flat-sequence {
            tunnel: w387 -> [w397]
            tunnel: [w397] -> w386
            frame #0 {
              n184 = Unbundle By Name(w397) -> ("pWVI"=w400:refnum<vi>)
              n185 = invoke class="VI" method="Ctrl Val.Set"(reference=w400, "Control Name"="sCloseMode", "Value"="NOSAVE" ("Control Name")) -> ()  [unwired: 2 in, 5 out]
            }
          }
          n186 = global read "CRYMain Sub Window Global.vi" "tWinType"() -> (w394:T7)
          n187 = Unbundle By Name(w394) -> ("CLOSE_CLOSE"=w388:i32, "DOCK_DISABLE"=w396:i32, "FOCUS_SHOW"=w395:i32)
          n188 = Compound Arithmetic op=OR(w388, w396, w395) -> (w393:i32)
          n189 = Bundle By Name(cluster=w386, "nProperty"=w393) -> (w391:T2)
          n190 = call "CRYAPI FRAME.vi"("tFrame"=w391, "sAction"="REPLACE_FRAME") -> ("tFrame_Out"=w389:T2)  [unwired: 6 in, 3 out]
          n191 = call "CRYAPI MANAGER.vi"("tFrame"=w389, "sAction"="CLOSE_VI") -> ()  [unwired: 3 in, 7 out]
        }
        frame 0 {
        }
      }
    }
    frame "CloseVI" {
      n192 = call "CRYAPI FRAME.vi"("sData"=w401, "sAction"="FIND_WIN") -> ("nData_Out"=w404:i32, "sData_Out"=w402:string, "tFrame_Out"=w403:T2)  [unwired: 4 in, 3 out]
      n193 = case shown="Default" w404 {
        tunnel: w403 -> [w406 _]
        tunnel: w402 -> [_ _]
        tunnel: w401 -> [w408 _]
        frame Default {
          n194 = case shown="\"Add Step\"" w408 {
            tunnel: [TRUE w412] -> w407
            tunnel: w406 -> [_ w418]
            frame Default {
            }
            frame "Add Step" {
              n195 = Unbundle By Name(w418) -> ("pVIW"=w417:refnum<vi>)
              n196 = invoke class="VI" method="Ctrl Val.Get"(reference=w417, "Control Name"="PinTrue") -> ("Get Control Value Variant"=w415:variant)  [unwired: 2 in, 3 out]
              n197 = Variant To Data(type=TRUE, Variant=w415) -> (data=w413:bool)  [unwired: 1 in, 1 out]
              n198 = Not(x=w413) -> (.not. x?=w412:bool)
            }
          }
          n199 = case shown="True" w407 {
            tunnel: w406 -> [_ w409]
            frame False {
            }
            frame True {
              n200 = call "CRYAPI MANAGER.vi"("tFrame"=w409, "sAction"="CLOSE_VI") -> ()  [unwired: 3 in, 7 out]
            }
          }
        }
        frame 0 {
        }
      }
    }
    frame "CLOSE_FRAME" {
      n201 = Decimal String To Number(string=w420) -> (number=w419:i32)  [unwired: 2 in, 1 out]
      n202 = call "CRYAPI DOCKING.vi"("nSWinID"=w419, "sAction"="CLOSE_FRAME") -> ()  [unwired: 2 in, 8 out]
    }
    frame "PROJECT_RUN", "PROJECT_STOP" {
      n203 = call "CRYPIC Change Sate.vi"("sAction"=w422) -> ("sData_Out"=w423:string)  [unwired: 10 in]
      n204 = case shown="\"PROJECT_RUN\"" w423 {
        frame "PROJECT_STOP", Default {
        }
        frame "PROJECT_RUN" {
          n205 = call "CRYAPI FRAME.vi"("sData"="Add Step", "sAction"="FIND_WIN") -> ("tFrame_Out"=w424:T2)  [unwired: 4 in, 5 out]
          n206 = Unbundle By Name(w424) -> ("pVIW"=w427:refnum<vi>)
          n207 = property class="VI"(reference=w427) -> (reference out=w425:refnum<vi>, "FP.State"=w426:T3)  [unwired: 1 in, 1 out]
          n208 = case shown="\"Standard\"" w426 {
            tunnel: w425 -> [_ w432]
            tunnel: w424 -> [_ w430]
            frame "Invalid", Default {
            }
            frame "Standard" {
              n209 = invoke class="VI" method="Ctrl Val.Set"(reference=w432, "Control Name"="PinTrue", "Value"=FALSE) -> (reference out=w431:refnum<vi>)  [unwired: 2 in, 4 out]
              n210 = flat-sequence {
                tunnel: w431 -> [_]
                tunnel: w430 -> [w435]
                frame #0 {
                  n211 = call "CRYAPI MANAGER.vi"("tFrame"=w435, "sAction"="CLOSE_VI") -> ()  [unwired: 3 in, 7 out]
                }
              }
            }
          }
        }
      }
    }
  }
